vi "Distribute 5-bar Torque.vi"(8 "error in (no error)":errorcluster, 10 "joint_torques":dbl[](array[numeric]), 11 "Finger in":refnum<class "Finger.lvclass">) -> (0 "error out":errorcluster, 2 "motor_torques":dbl[](array[numeric]), 3 "Finger out":refnum<class "Finger.lvclass">)   [LabVIEW 2013, in "Finger.lvclass"]
uses:
  Finger.lvclass
  Finger.lvclass/Finger.ctl
  <vilib>/Analysis/Matrix/Datatypes/RealMatrix.ctl
  <vilib>/Analysis/Matrix/Numeric/Multiply/Multiply - RM,RM.vi
  <vilib>/Analysis/Matrix/Numeric/Conversions/Array To Matrix - RA.vi
  <vilib>/Analysis/Matrix/NI_Matrix.lvlib
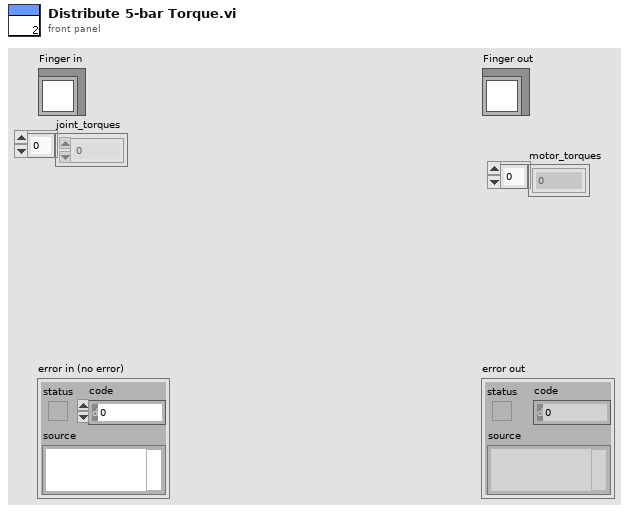
[diagram p1: front panel]
types:
  T1 = typedef "NI_Matrix.lvlib/RealMatrix.ctl" = dbl[][]
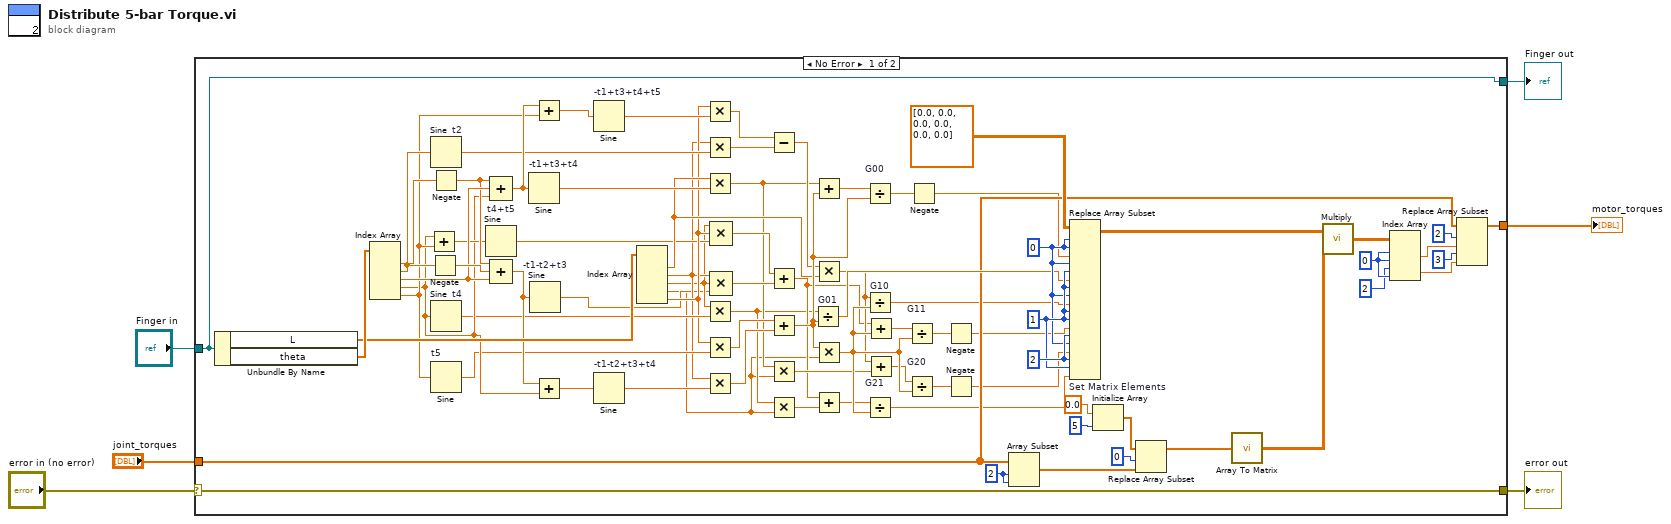
[diagram p0: block diagram]
diagram:
  n1 = case shown="No Error" "error in (no error)" {
    selector: "error in (no error)" -> [w85 w87]
    tunnel: [w85 w87] -> w5
    tunnel: [w84 w86] -> w3
    tunnel: "Finger in" -> [w84 w86]
    tunnel: [w83 _] -> w1
    tunnel: "joint_torques" -> [w49 _]
    frame No Error {
      w41 = 0 ("index (row)")
      w59 = 2 ("disabled index (row)")
      w58 = 1 ("disabled index (row)")
      w57 = 0 ("disabled index (row)")
      w50 = 2 ("index")
      n2 = Unbundle By Name(w84) -> ("L"=w79:dbl[], "theta"=w80:dbl[])
      n3 = Index Array(array=w80) -> (element #1=w78:dbl, element #2=w72:dbl, element #3=w76:dbl, element #4=w68:dbl, element #5=w71:dbl)  [unwired: 5 in]
      n4 = Add(x=w68, y=w71) -> (x+y=w70:dbl)
      n5 = Negate(x=w72) -> (-x=w77:dbl)
      n6 = Sine "t2"(x=w72) -> (sin(x)=w25:dbl)
      n7 = Negate(x=w78) -> (-x=w75:dbl)
      n8 = Sine "t4"(x=w68) -> (sin(x)=w60:dbl)
      n9 = Sine "t5"(x=w71) -> (sin(x)=w66:dbl)
      n10 = Sine "t4+t5"(x=w70) -> (sin(x)=w19:dbl)
      n11 = Compound Arithmetic op=ADD(w75, w76, w68) -> (w74:dbl)
      n12 = Compound Arithmetic op=ADD(w75, w77, w76) -> (w69:dbl)
      n13 = Sine "-t1+t3+t4"(x=w74) -> (sin(x)=w62:dbl)
      n14 = Sine "-t1-t2+t3"(x=w69) -> (sin(x)=w16:dbl)
      n15 = Add(x=w74, y=w71) -> (x+y=w73:dbl)
      n16 = Add(x=w69, y=w68) -> (x+y=w67:dbl)
      n17 = Sine "-t1+t3+t4+t5"(x=w73) -> (sin(x)=w37:dbl)
      n18 = Sine "-t1-t2+t3+t4"(x=w67) -> (sin(x)=w65:dbl)
      n19 = Index Array(array=w79) -> (element #1=w27:dbl, element #2=w18:dbl, element #3=w17:dbl, element #4=w7:dbl, element #5=w20:dbl)  [unwired: 5 in]
      n20 = Multiply(x=w20, y=w37) -> (x*y=w36:dbl)
      n21 = Multiply(x=w18, y=w25) -> (x*y=w26:dbl)
      n22 = Multiply(x=w27, y=w62) -> (x*y=w14:dbl)
      n23 = Multiply(x=w17, y=w60) -> (x*y=w8:dbl)
      n24 = Multiply(x=w20, y=w66) -> (x*y=w63:dbl)
      n25 = Multiply(x=w18, y=w65) -> (x*y=w64:dbl)
      n26 = Compound Arithmetic op=MULTIPLY(w17, w20, w19) -> (w21:dbl)
      n27 = Compound Arithmetic op=MULTIPLY(w18, w17, w16) -> (w22:dbl)
      n28 = Subtract(x=w36, y=w26) -> (x-y=w28:dbl)
      n29 = Add(x=w21, y=w22) -> (x+y=w10:dbl)
      n30 = Add(x=w63, y=w64) -> (x+y=w39:dbl)
      n31 = Multiply(x=w14, y=w7) -> (x*y=w13:dbl)
      n32 = Multiply(x=w8, y=w7) -> (x*y=w9:dbl)
      n33 = Divide "G01"(x=w8, y=w39) -> (x/y=w55:dbl)
      n34 = Add(x=w14, y=w39) -> (x+y=w61:dbl)
      n35 = Multiply(x=w28, y=w27) -> (x*y=w15:dbl)
      n36 = Multiply(x=w39, y=w7) -> (x*y=w23:dbl)
      n37 = Add(x=w10, y=w9) -> (x+y=w11:dbl)
      n38 = Divide "G00"(x=w61, y=w39) -> (x/y=w35:dbl)
      n39 = Divide "G10"(x=w15, y=w23) -> (x/y=w38:dbl)
      n40 = Divide "G21"(x=w11, y=w23) -> (x/y=w29:dbl)
      n41 = Add(x=w10, y=w23) -> (x+y=w24:dbl)
      n42 = Add(x=w15, y=w13) -> (x+y=w12:dbl)
      n43 = Divide "G11"(x=w24, y=w23) -> (x/y=w33:dbl)
      n44 = Divide "G20"(x=w12, y=w23) -> (x/y=w32:dbl)
      n45 = Negate(x=w35) -> (-x=w34:dbl)
      n46 = Negate(x=w33) -> (-x=w31:dbl)
      n47 = Negate(x=w32) -> (-x=w30:dbl)
      n48 = Array Subset(array=w49, index=w50, length=w50) -> (w48:dbl[])
      n49 = Replace Array Subset "Set Matrix Elements"(array=T1 [[0.0, 0.0], [0.0, 0.0], [0.0, 0.0]] ("output matrix"), new element #1=w34, index (row) #1=w57, index (col) #1=w57, new element #2=w55, index (row) #2=w57, index (col) #2=w58, new element #3=w38, index (row) #3=w58, index (col) #3=w57, new element #4=w31, index (row) #4=w58, index (col) #4=w58, new element #5=w30, index (row) #5=w59, index (col) #5=w57, new element #6=w29, index (row) #6=w59, index (col) #6=w58) -> (w47:T1)
      n50 = Initialize Array(0.0 ("element"), 5 ("dimension size")) -> (w51:dbl[])
      n51 = Replace Array Subset(array=w51, new element=w48, index=0) -> (w46:dbl[])
      n52 = call-poly <vilib>:"Array To Matrix.vi"("Real 1D Array"=w46) -> ("Real Matrix (Column Vector)"=w45:T1)
      n53 = call-poly <vilib>:"Multiply.vi"("Real Matrix B"=w45, "Real Matrix A"=w47) -> ("A * B"=w42:T1)
      n54 = Index Array(array=w42, index (row) #1=w41, index (col) #1=w41, index (row) #2=2 ("disabled index (row)"), index (col) #2=w41) -> (element #1=w44:dbl, element #2=w43:dbl)
      n55 = Replace Array Subset(array=w49, new element #1=w44, index #1=2 ("index"), new element #2=w43, index #2=3 ("index")) -> (w83:dbl[])
    }
    frame Error {
    }
  }
  "error out" <- w5
  "Finger out" <- w3
  "motor_torques" <- w1
